vi "Generate Drain Report Text.vi"(0 "Drain State DAQ In":bool[](array[boolean]), 11 "Drain State ERD In":string[](array[string])) -> (4 "Pass/Fail?":bool, 15 "Report Text":string)   [LabVIEW 2016, in "TLMB.lvlib"]
uses:
  Projects/TLMB.lvlib
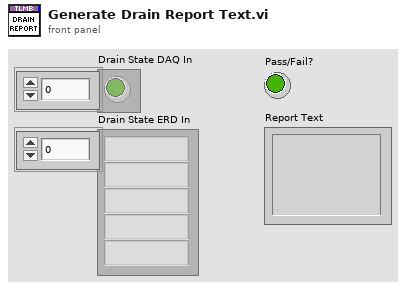
[diagram p1: front panel]
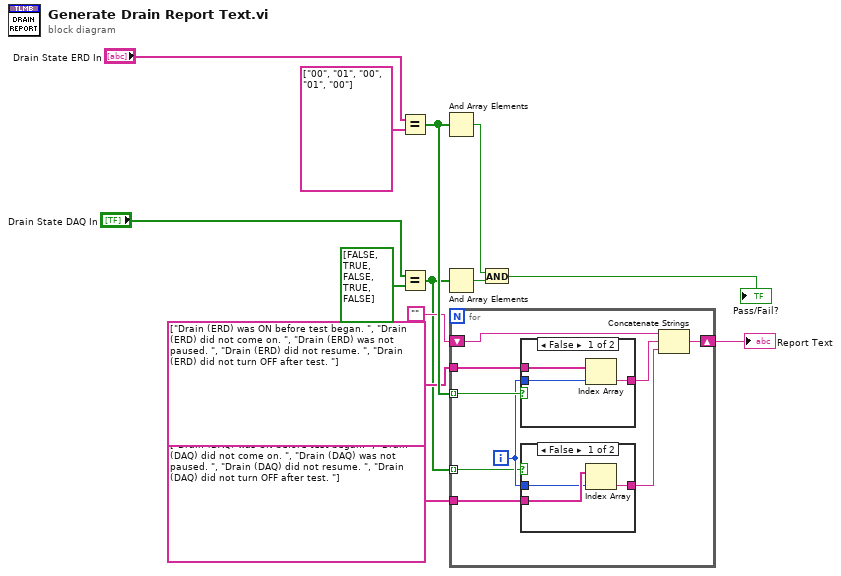
[diagram p0: block diagram]
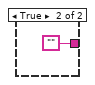
[diagram p2: hidden frame]
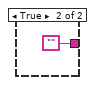
[diagram p3: hidden frame]
diagram:
  n1 = Equal?(x="Drain State ERD In", y=string[] ["00", "01", "00", "01", "00"]) -> (x = y?=w8:bool[])
  n2 = Equal?(x="Drain State DAQ In", y=bool[] [FALSE, TRUE, FALSE, TRUE, FALSE]) -> (x = y?=w3:bool[])
  n3 = And Array Elements(Boolean array=w8) -> (logical AND=w9:bool)
  n4 = And Array Elements(Boolean array=w3) -> (logical AND=w11:bool)
  n5 = for {
    tunnel: w8 -> [w22] mode=indexing
    tunnel: string[] ["Drain (ERD) was ON before test began. ", "Drain (ERD) did not come on. ", "Drain (ERD) was not paused. ", "Drain (ERD) did not resume. ", "Drain (ERD) did not turn OFF after test. "] ("y") -> [w21]
    shift-right: [w18] -> w2
    shift-left: "" -> [w20]
    tunnel: string[] ["Drain (DAQ) was ON before test began. ", "Drain (DAQ) did not come on. ", "Drain (DAQ) was not paused. ", "Drain (DAQ) did not resume. ", "Drain (DAQ) did not turn OFF after test. "] ("y") -> [w17]
    tunnel: w3 -> [w14] mode=indexing
    i -> [w16]
    n6 = case shown="False" w22 {
      tunnel: w21 -> [w29 _]
      tunnel: w16 -> [w28 _]
      tunnel: [w27 ""] -> w19
      frame False {
        n7 = Index Array(array=w29, index=w28) -> (element=w27:string)
      }
      frame True {
      }
    }
    n8 = case shown="False" w14 {
      tunnel: w17 -> [w25 _]
      tunnel: w16 -> [w24 _]
      tunnel: [w23 ""] -> w15
      frame False {
        n9 = Index Array(array=w25, index=w24) -> (element=w23:string)
      }
      frame True {
      }
    }
    n10 = Concatenate Strings(w20, w19, w15) -> (w18:string)
  }
  "Report Text" <- w2
  n11 = And(x=w9, y=w11) -> (x .and. y?=→"Pass/Fail?":bool)
